vi "Set_Parameter_Instrument (Json).vi"(8 "error in (no error)":errorcluster caption="entrée d'erreur (pas d'erreur)", 10 "Parameter (Json)":string, 11 "Flash_SIN_FP en entrée":refnum<class "Get_Mac_Addr.lvclass">) -> (0 "error out":errorcluster caption="sortie d'erreur", 3 "Flash_SIN_FP en sortie":refnum<class "Get_Mac_Addr.lvclass">)   [LabVIEW 2020, in "Library Test.lvlib" / "Get_Mac_Addr.lvclass"]
uses:
  Get_Mac_Addr.lvclass
  C:/Users/ngarcin/OneDrive - Altyor/Standard TB/Class/Test/Test (Default)/Test (Default).lvclass
  C:/Users/ngarcin/OneDrive - Altyor/Standard TB/Class/Test/Flash_Commander/Flash_Commander.lvclass
  Get_Mac_Addr.lvclass/Get_Mac_Addr.ctl
  JSON API/JSON Value/Set from JSON string.vi
  Flash_Commander/Flash_Commander.lvclass
  JSON API/JSON Value/JSON Value.lvclass
  JSON API/Variant JSON/Variant JSON.lvlib
  JSON API/Get Polymorphic/JSON GetSet.lvlib
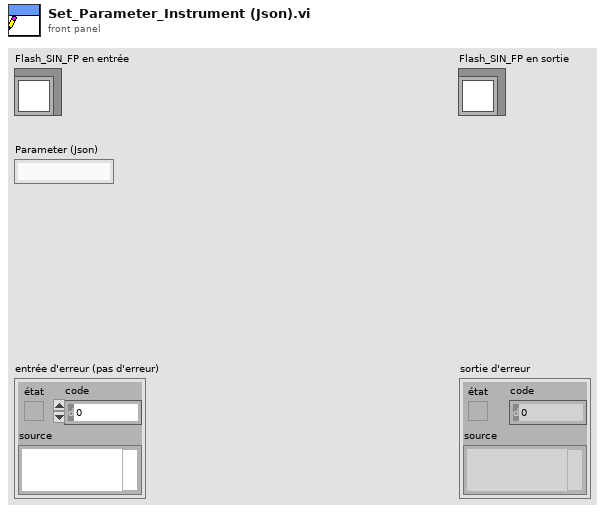
[diagram p1: front panel]
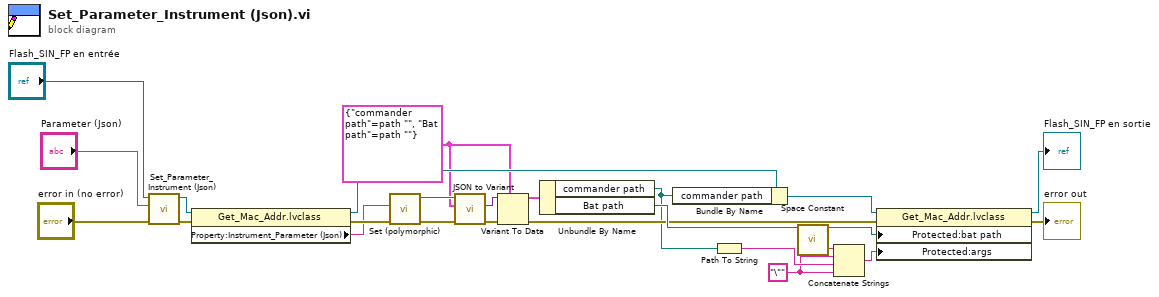
[diagram p0: block diagram]
diagram:
  w1 = "\""
  w11 = cluster{"commander path":path, "Bat path":path} {"commander path"=path "", "Bat path"=path ""} ("Cluster des données privées de classe")
  n1 = call-parent "Set_Parameter_Instrument (Json).vi"("error in (no error)"="error in (no error)", "Parameter (Json)"="Parameter (Json)", "Test (Default) en entrée"="Flash_SIN_FP en entrée") -> ("error out"=w19:errorcluster, "Test (Default) en sortie"=w18:refnum<class "Get_Mac_Addr.lvclass">)  [unwired: 7 in]
  n2 = property class="Get_Mac_Addr.lvclass"(reference=w18, error in=w19) -> (reference out=w14:refnum<class "Get_Mac_Addr.lvclass">, error out=w17:errorcluster, "Property:Instrument_Parameter (Json)"=w15:string)
  n3 = call-poly "Set (polymorphic).vi"("error in (no error)"=w17, "JSON stream"=w15) -> ("error out"=w22:errorcluster, "JSON Value out"=w24:refnum<class "JSON Value.lvclass">)  [unwired: 7 in, 1 out]
  n4 = call "JSON to Variant.vi"("error in (no error)"=w22, "Variant (Data Type)"=w11, "JSON Value"=w24) -> ("error out"=w23:errorcluster, "Variant out"=w21:variant)  [unwired: 7 in]
  n5 = Variant To Data(error in=w23, type=w11, Variant=w21) -> (data=w13:cluster{"commander path":path, "Bat path":path}, error out=w3:errorcluster)
  n6 = Unbundle By Name(w13) -> ("commander path"=w2:path, "Bat path"=w5:path)
  n7 = Bundle By Name(cluster=w14, "commander path"=w2) -> (w10:refnum<class "Get_Mac_Addr.lvclass">)
  n8 = Path To String(path=w2) -> (string=w6:string)
  n9 = call <vilib>:"Space Constant.vi"() -> ("String"=w7:string)
  n10 = Concatenate Strings(w7, w1, w6, w1) -> (w4:string)
  n11 = property class="Get_Mac_Addr.lvclass"(reference=w10, error in=w3, "Protected:bat path"=w5, "Protected:args"=w4) -> (reference out=→"Flash_SIN_FP en sortie":refnum<class "Get_Mac_Addr.lvclass">, error out=→"error out":errorcluster)
